vi "Actor Core.vi"(8 "error in":errorcluster, 11 "lightfield_panel in":refnum<class "lightfield_panel.lvclass">) -> (0 "error out":errorcluster, 3 "Actor out":refnum<class "Actor.lvclass">)   [LabVIEW 2015, in "lightfield_panel.lvclass"]
doc: "(<B>Filename</B>: Actor Framework.lvlib:Actor.lvclass:Actor Core.vi)\n\nReceives messages to the actor, reacts to them, and initiates any error handling that may shut the actor down.\n\nDescendant classes may override this VI to append parallel tasks for the actor to complete while it handles messages. Overrides use the Call Parent Method node."
uses:
  lightfield_panel.lvclass
  <vilib>/ActorFramework/Actor/Actor.lvclass
  lfield_settings.ctl
  UI/panel_class/panel.lvclass/panel.ctl
  <vilib>/ActorFramework/Actor/Actor.lvclass/Actor.ctl
  <vilib>/ActorFramework/Message Enqueuer/Message Enqueuer.lvclass/Message Enqueuer.ctl
  lightfield_panel Messages/lfieldpanel_connect Msg/lfieldpanel_connect Msg.lvclass/lfieldpanel_connect Msg.ctl
  lightfield_panel Messages/lfieldpanel_set_experiment Msg/lfieldpanel_set_experiment Msg.lvclass/lfieldpanel_set_experiment Msg.ctl
  lightfield_panel Messages/lfieldpanel_acquire_single_frame Msg/lfieldpanel_acquire_single_frame Msg.lvclass/lfieldpanel_acquire_single_frame Msg.ctl
  lightfield_panel Messages/lfieldpanel_stream_frames Msg/lfieldpanel_stream_frames Msg.lvclass/lfieldpanel_stream_frames Msg.ctl
  lightfield_panel Messages/lfieldpanel_dynamic_subtraction Msg/lfieldpanel_dynamic_subtraction Msg.lvclass/lfieldpanel_dynamic_subtraction Msg.ctl
  Stage Class/thorlabs_filter_wheel/thorlabs_FW102C.lvclass
  <vilib>/ActorFramework/Message Enqueuer/Init from Existing Queue.vi
  <vilib>/ActorFramework/Message Enqueuer/Enqueue.vi
  <vilib>/ActorFramework/Message Priority Queue/Priority Enqueue.vi
  <vilib>/ActorFramework/Message Enqueuer/Message Enqueuer.lvclass
  lightfield_panel Messages/lfieldpanel_disconnect Msg/lfieldpanel_disconnect Msg.lvclass
  lightfield_panel Messages/lfieldpanel_connect Msg/lfieldpanel_connect Msg.lvclass
  lightfield_panel Messages/lfieldpanel_set_experiment Msg/lfieldpanel_set_experiment Msg.lvclass
  lightfield_panel Messages/lfieldpanel_acquire_single_frame Msg/lfieldpanel_acquire_single_frame Msg.lvclass
  lightfield_panel Messages/lfieldpanel_stream_frames Msg/lfieldpanel_stream_frames Msg.lvclass
  lightfield_panel Messages/lfieldpanel_dynamic_subtraction Msg/lfieldpanel_dynamic_subtraction Msg.lvclass
  UI/panel_class/panel.lvclass
panel:
  in  "dynamic_backg":bool
  in  "Integrate Sensor Area":bool
  in  "stream_frames":bool
  in  "Open Lightfield?":bool=TRUE
  in  "acq_1_frame":bool
  in  "lfield_settings_tab":enum32{"Basic Settings"}(tab)
  in  "shutter_control":bool
  in  "Notes":string
  in  "Number of Frames":i32
  in  "Log Data":bool
  in  "Save Path":path
  in  "Experiment Name":string(combo)
  in  "Lightfield Settings":T1
  in  "set_experiment":bool
  out "Status":string
  in  "connect_lightfield":bool
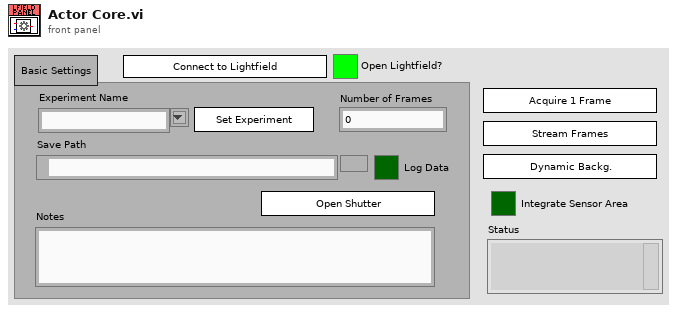
[diagram p1: front panel]
types:
  T1 = typedef "lfield_settings.ctl" = cluster{"Exposure (s)":dbl, "Avg. Frames":dbl}
  T2 = typedef "lfield_ui_event_refs.ctl" = cluster{"update_lfield_status":refnum<event-registration>, "update_experiment_names":refnum<event-registration>, "plot_1d_data":refnum<event-registration>, "plot_2d_data":refnum<event-registration>, "chart_0d_data":refnum<event-registration>}
  T3 = cluster{"update_lfield_status":refnum<event-registration>, "stop_ui_ref":refnum<event-registration>, "update_experiment_names":refnum<event-registration>}
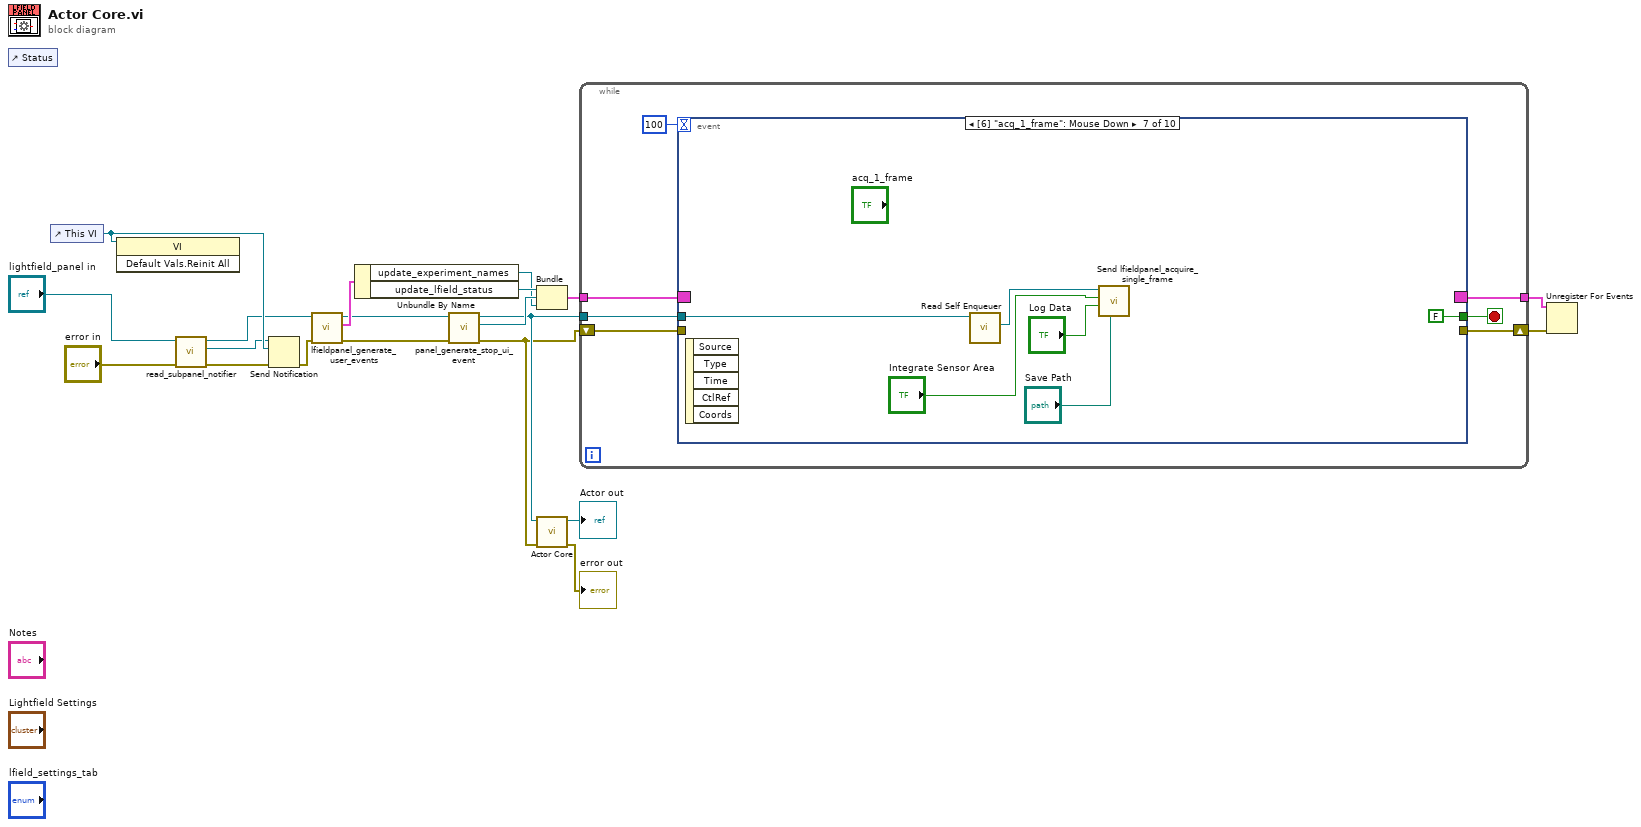
[diagram p0: block diagram]
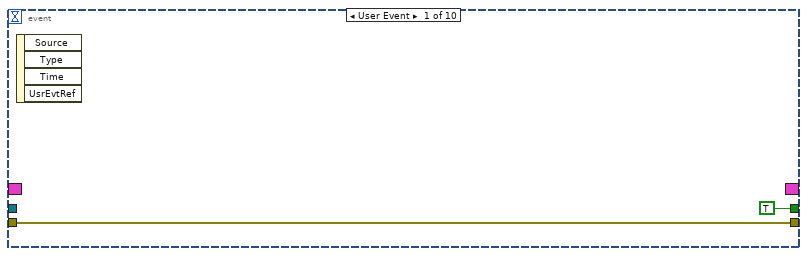
[diagram p2: hidden frame]
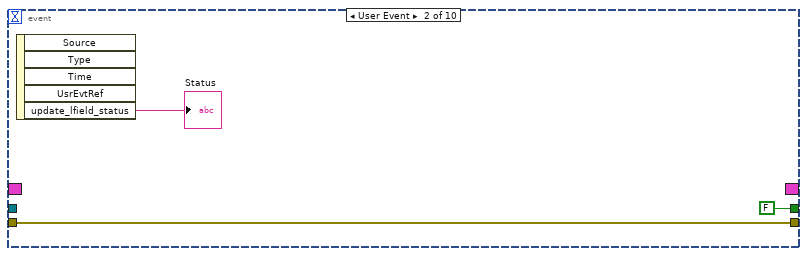
[diagram p3: hidden frame]
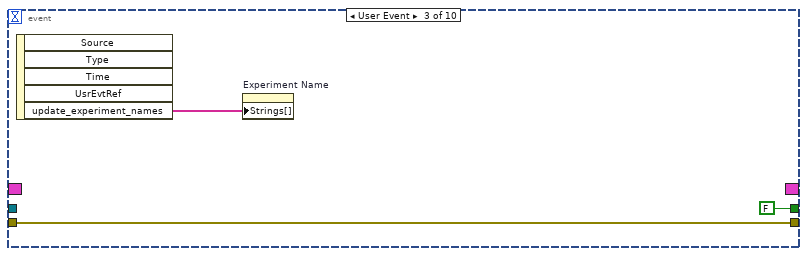
[diagram p4: hidden frame]
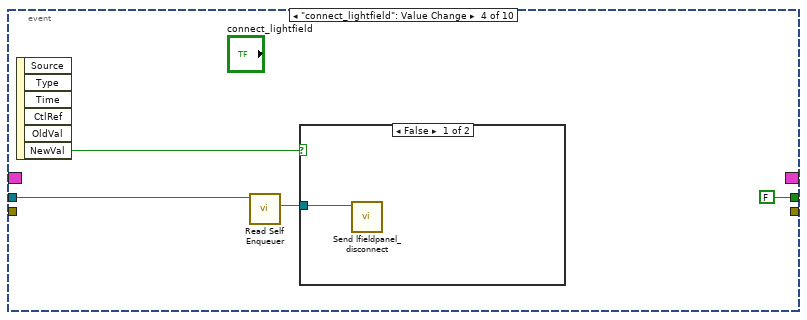
[diagram p5: hidden frame]
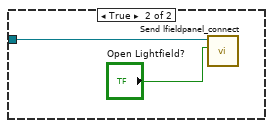
[diagram p6: hidden frame]
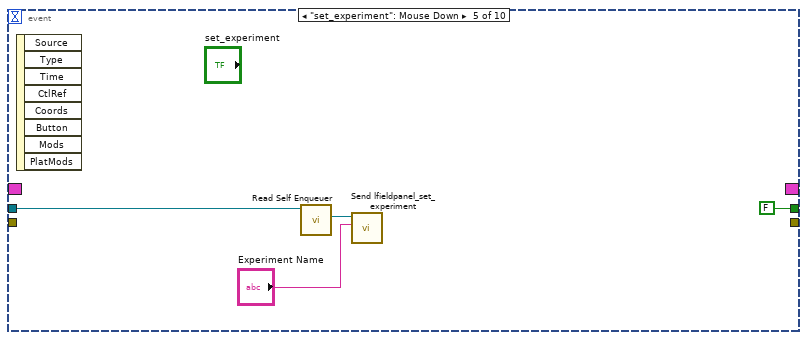
[diagram p7: hidden frame]
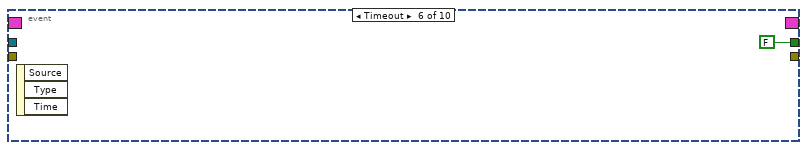
[diagram p8: hidden frame]
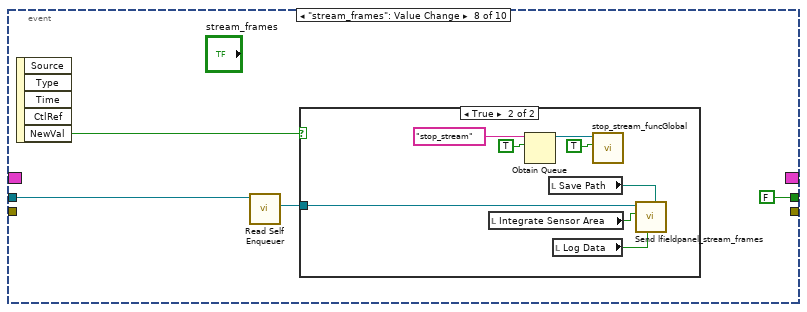
[diagram p9: hidden frame]
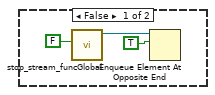
[diagram p10: hidden frame]
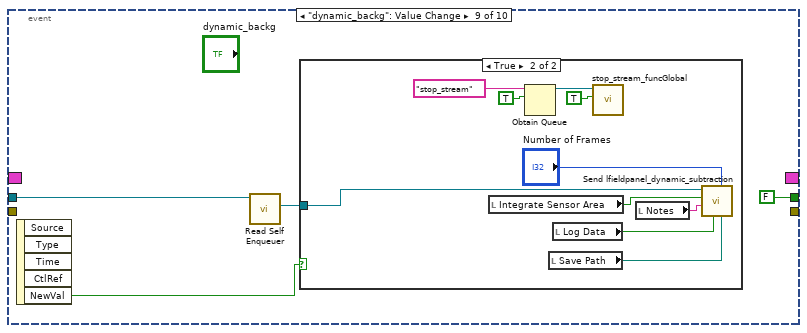
[diagram p11: hidden frame]
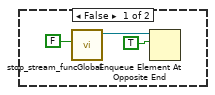
[diagram p12: hidden frame]
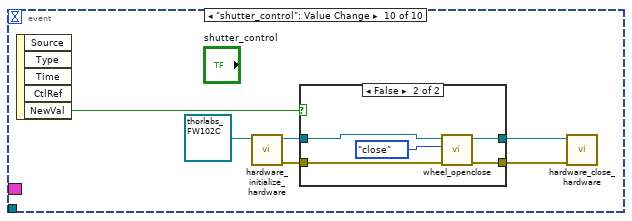
[diagram p13: hidden frame]
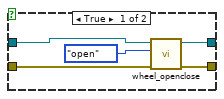
[diagram p14: hidden frame]
diagram:
  n1 = control-ref of="Status"() -> ()  [unwired: 1 out]
  n2 = control-ref of="This VI"() -> (w17:refnum<vi>)
  n3 = invoke class="VI" method="Default Vals.Reinit All"(reference=w17) -> ()  [unwired: 2 in, 3 out]
  n4 = call "read_subpanel_notifier.vi"("error in (no error)"="error in", "panel in"="lightfield_panel in") -> ("error out"=w3:errorcluster, "subpanel_notifier"=w13:refnum<notifier>, "panel out"=w5:refnum<class "lightfield_panel.lvclass">)  [unwired: 7 in]
  n5 = Send Notification(notification=w17, notifier=w13, error in (no error)=w3) -> (error out=w12:errorcluster)  [unwired: 1 out]
  n6 = call "lfieldpanel_generate_user_events.vi"("error in (no error)"=w12, "lightfield_panel in"=w5) -> ("error out"=w11:errorcluster, "lfield_ui_events"=w10:T2, "lightfield_panel out"=w9:refnum<class "lightfield_panel.lvclass">)  [unwired: 7 in]
  n7 = Unbundle By Name(w10) -> ("update_experiment_names"=w1:refnum<event-registration>, "update_lfield_status"=w15:refnum<event-registration>)
  n8 = call "panel_generate_stop_ui_event.vi"("error in (no error)"=w11, "panel in"=w9) -> ("error out"=w7:errorcluster, "stop_ui_ref"=w16:refnum<event-registration>, "panel out"=w8:refnum<class "lightfield_panel.lvclass">)  [unwired: 7 in]
  n9 = Bundle("update_lfield_status"=w15, "stop_ui_ref"=w16, "update_experiment_names"=w1) -> (w14:T3)  [unwired: 1 in]
  n10 = call-parent "Actor Core.vi"("error in"=w7, "Actor in"=w8) -> ("error out"=→"error out":errorcluster, "Actor out"=→"Actor out":refnum<class "Actor.lvclass">)  [unwired: 8 in]
  n11 = while {
    tunnel: [w27] -> w2
    shift-right: [w24] -> w18
    shift-left: w7 -> [w25]
    tunnel: w8 -> [w23]
    tunnel: w14 -> [w21]
    stop <- w26 stop-if-true
    n12 = event shown="[6] \"acq_1_frame\": Mouse Down" {
      selector: w21 -> [_ _ _ _ _ _ _ _ _ _]
      dyn-events: [_ _ _ _ _ _ _ _ _ _] -> w27
      timeout: 100 -> [_ _ _ _ _ _ _ _ _ _]
      tunnel: [TRUE FALSE FALSE FALSE FALSE FALSE FALSE FALSE FALSE _] -> w26
      tunnel: w25 -> [w28 w30 w33 _ _ _ _ _ _ _]
      tunnel: [w28 w30 w33 _ _ _ _ _ _ _] -> w24
      tunnel: w23 -> [_ _ _ w37 w46 _ w53 w55 w70 _]
      event User Event {
        n13 = event-data() -> ()  [unwired: 1 in, 4 out]
      }
      event User Event {
        n14 = event-data() -> ("update_lfield_status"=→"Status":string)  [unwired: 1 in, 4 out]
      }
      event User Event {
        n15 = event-data() -> ("update_experiment_names"=w35:string[])  [unwired: 1 in, 4 out]
        n16 = property on="Experiment Name" class="CmbBox"("Strings[]"=w35) -> ()  [unwired: 2 in, 2 out]
      }
      event "connect_lightfield": Value Change {
        n17 = event-data() -> ("NewVal"=w39:bool)  [unwired: 1 in, 5 out]
        n18 = call <vilib>:"Read Self Enqueuer.vi"("Actor"=w37) -> ("Self Enqueuer"=w36:refnum<class "Message Enqueuer.lvclass">)  [unwired: 10 in]
        n19 = case shown="False" w39 {
          tunnel: w36 -> [w40 w42]
          frame False {
            n20 = call "Send lfieldpanel_disconnect.vi"("Message Enqueuer"=w40) -> ()  [unwired: 9 in, 2 out]
          }
          frame True {
            n21 = call "Send lfieldpanel_connect.vi"("Is Visible?"="Open Lightfield?", "Message Enqueuer"=w42) -> ()  [unwired: 8 in, 2 out]
          }
        }
      }
      event "set_experiment": Mouse Down {
        n22 = event-data() -> ()  [unwired: 1 in, 8 out]
        n23 = call <vilib>:"Read Self Enqueuer.vi"("Actor"=w46) -> ("Self Enqueuer"=w45:refnum<class "Message Enqueuer.lvclass">)  [unwired: 10 in]
        n24 = call "Send lfieldpanel_set_experiment.vi"("experiment_name"="Experiment Name", "Message Enqueuer"=w45) -> ()  [unwired: 8 in, 2 out]
      }
      event Timeout {
        n25 = event-data() -> ()  [unwired: 1 in, 3 out]
      }
      event "acq_1_frame": Mouse Down {
        n26 = event-data() -> ()  [unwired: 1 in, 5 out]
        n27 = call <vilib>:"Read Self Enqueuer.vi"("Actor"=w53) -> ("Self Enqueuer"=w52:refnum<class "Message Enqueuer.lvclass">)  [unwired: 10 in]
        n28 = call "Send lfieldpanel_acquire_single_frame.vi"("savepath"="Save Path", "Log data"="Log Data", "Integrate_sensor"="Integrate Sensor Area", "Message Enqueuer"=w52) -> ()  [unwired: 6 in, 2 out]
      }
      event "stream_frames": Value Change {
        n29 = event-data() -> ("NewVal"=w57:bool)  [unwired: 1 in, 4 out]
        n30 = call <vilib>:"Read Self Enqueuer.vi"("Actor"=w55) -> ("Self Enqueuer"=w54:refnum<class "Message Enqueuer.lvclass">)  [unwired: 10 in]
        n31 = case shown="True" w57 {
          tunnel: w54 -> [_ w68]
          frame False {
            n32 = call "stop_stream_funcGlobal.vi"("write?"=FALSE) -> ("queue out 2"=w59:refnum<queue>)  [unwired: 10 in]
            n33 = Enqueue Element At Opposite End(queue=w59, element=TRUE) -> ()  [unwired: 2 in, 3 out]
          }
          frame True {
            n34 = local read "Integrate Sensor Area"() -> (w67:bool)
            n35 = Obtain Queue(name (unnamed)="stop_stream", element data type=TRUE) -> (queue out=w61:refnum<queue>)  [unwired: 3 in, 2 out]
            n36 = local read "Save Path"() -> (w66:path)
            n37 = local read "Log Data"() -> (w65:bool)
            n38 = call "stop_stream_funcGlobal.vi"("write?"=TRUE, "queue out"=w61) -> ()  [unwired: 9 in, 1 out]
            n39 = call "Send lfieldpanel_stream_frames.vi"("savepath"=w66, "Log data"=w65, "Integrate_sensor"=w67, "Message Enqueuer"=w68) -> ()  [unwired: 6 in, 2 out]
          }
        }
      }
      event "dynamic_backg": Value Change {
        n40 = event-data() -> ("NewVal"=w72:bool)  [unwired: 1 in, 4 out]
        n41 = call <vilib>:"Read Self Enqueuer.vi"("Actor"=w70) -> ("Self Enqueuer"=w69:refnum<class "Message Enqueuer.lvclass">)  [unwired: 10 in]
        n42 = case shown="True" w72 {
          tunnel: w69 -> [_ w81]
          frame False {
            n43 = call "stop_stream_funcGlobal.vi"("write?"=FALSE) -> ("queue out 2"=w74:refnum<queue>)  [unwired: 10 in]
            n44 = Enqueue Element At Opposite End(queue=w74, element=TRUE) -> ()  [unwired: 2 in, 3 out]
          }
          frame True {
            n45 = local read "Integrate Sensor Area"() -> (w79:bool)
            n46 = Obtain Queue(name (unnamed)="stop_stream", element data type=TRUE) -> (queue out=w82:refnum<queue>)  [unwired: 3 in, 2 out]
            n47 = local read "Save Path"() -> (w80:path)
            n48 = local read "Log Data"() -> (w77:bool)
            n49 = call "stop_stream_funcGlobal.vi"("write?"=TRUE, "queue out"=w82) -> ()  [unwired: 9 in, 1 out]
            n50 = local read "Notes"() -> (w78:string)
            n51 = call "Send lfieldpanel_dynamic_subtraction.vi"("savepath"=w80, "num_frames"="Number of Frames", "Log data"=w77, "notes"=w78, "Integrate_sensor"=w79, "Message Enqueuer"=w81) -> ()  [unwired: 4 in, 2 out]
          }
        }
      }
      event "shutter_control": Value Change {
        n52 = event-data() -> ("NewVal"=w90:bool)  [unwired: 1 in, 4 out]
        n53 = call-dynamic "hardware_initialize_hardware.vi"("thorlabs_FW102C in"=refnum<class "thorlabs_FW102C.lvclass"> refnum) -> ("error out"=w87:errorcluster, "thorlabs_FW102C out"=w89:refnum<class "thorlabs_FW102C.lvclass">)  [unwired: 9 in]
        n54 = case shown="False" w90 {
          tunnel: w89 -> [w96 w101]
          tunnel: [w95 w100] -> w88
          tunnel: w87 -> [w94 w99]
          tunnel: [w93 w98] -> w86
          frame True {
            n55 = call "wheel_openclose.vi"("error in (no error)"=w94, "action"=enum16{"open", "close"}."open", "thorlabs_FW102C in"=w96) -> ("error out"=w93:errorcluster, "thorlabs_FW102C out"=w95:refnum<class "thorlabs_FW102C.lvclass">)  [unwired: 7 in]
          }
          frame False {
            n56 = call "wheel_openclose.vi"("error in (no error)"=w99, "action"=enum16{"open", "close"}."close", "thorlabs_FW102C in"=w101) -> ("error out"=w98:errorcluster, "thorlabs_FW102C out"=w100:refnum<class "thorlabs_FW102C.lvclass">)  [unwired: 7 in]
          }
        }
        n57 = call-dynamic "hardware_close_hardware.vi"("error in (no error)"=w86, "thorlabs_FW102C in"=w88) -> ()  [unwired: 8 in, 2 out]
      }
    }
  }
  n58 = Unregister For Events(event registration refnum=w2, error in=w18) -> ()  [unwired: 1 out]
